vi "ErrorHandling.addLastErrorToFile.vi"(0 "ErrorHandling in":refnum<class "ErrorHandling.lvclass">, 5 "error in (no error)":errorcluster) -> (14 "ErrorHandling out":refnum<class "ErrorHandling.lvclass">, 19 "error out":errorcluster)   [LabVIEW 2016, in "ErrorHandling.lvclass"]
doc: "Schreibt das letzte Error-Ereignis in das entsprechende \"ErrorFile\" gem. System Pfadeintrag\n\n15.04.14 / sige"
uses:
  ErrorHandling.lvclass
  ErrorHandling.lvclass/ErrorHandling.ctl
  <vilib>/dlg_ctls.llb/Space Constant.vi
  <vilib>/Utility/error.llb/Trim Whitespace.vi
  <vilib>/Utility/error.llb/Search and Replace Pattern.vi
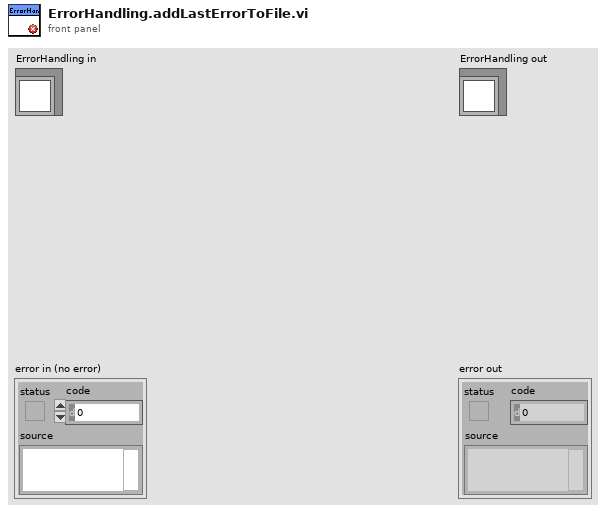
[diagram p1: front panel]
types:
  T1 = enum16{"open", "replace", "create", "open or create", "replace or create", "replace or create with confirmation"}
  T2 = typedef "ErrorHandling.lvclass/ErrorHandling.OccurredErrorDataStruct.ctl" = cluster{"Error":errorcluster, "Caller":string, "Comment":string, "Timestamp":timestamp, "Stopped":bool, "ErrorCusterString":string, "ErrorIndex":u64}
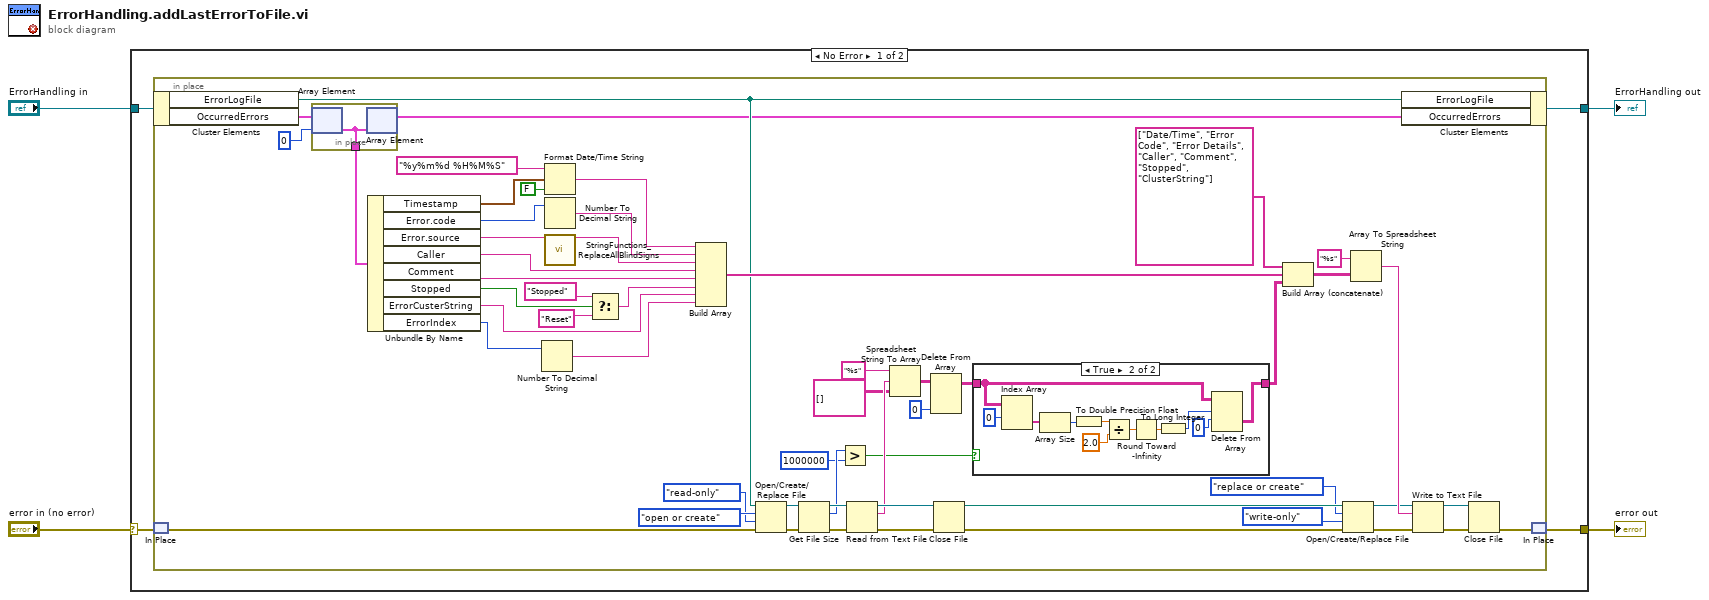
[diagram p0: block diagram]
diagram:
  n1 = case shown="No Error" "error in (no error)" {
    selector: "error in (no error)" -> [w7 w78]
    tunnel: [w6 w78] -> w3
    tunnel: [w5 w77] -> w1
    tunnel: "ErrorHandling in" -> [w8 w77]
    frame No Error {
      n2 = in-place {
        n3 = in-place-cluster #1(w8) -> ("ErrorLogFile"=w13:path, "OccurredErrors"=w12:T2[])
        n4 = in-place-match #2(w7) -> (w15:errorcluster)
        n5 = in-place {
          in-place-border: [w64] -> w11
          n6 = in-place-array #3(w12, 0) -> (w64:T2)
          n7 = in-place-array #3(w64) -> (w10:T2[])  [unwired: 1 out]
        }
        n8 = Unbundle By Name(w11) -> ("Timestamp"=w60:timestamp, "Error.code"=w63:i32, "Error.source"=w21:string, "Caller"=w19:string, "Comment"=w54:string, "Stopped"=w59:bool, "ErrorCusterString"=w18:string, "ErrorIndex"=w17:u64)
        n9 = Number To Decimal String(number=w17) -> (decimal integer string=w16:string)  [unwired: 1 in]
        n10 = Format Date/Time String(time format string (%c)="%y%m%d %H%M%S", seconds (now)=w60, UTC format=FALSE) -> (date/time string=w56:string)
        n11 = Number To Decimal String(number=w63) -> (decimal integer string=w55:string)  [unwired: 1 in]
        n12 = call "StringFunctions_ReplaceAllBlindSigns.vi"("String"=w21) -> ("ModifiedString"=w20:string)  [unwired: 17 in, 1 out]
        n13 = Select(t="Stopped", s=w59, f="Reset") -> (s? t:f=w53:string)
        n14 = Build Array(w56, w55, w20, w19, w54, w53, w18, w16) -> (w36:string[])
        n15 = Open/Create/Replace File(file path (use dialog)=w13, error in=w15, operation (0:open)=T1."open or create", access (0:read/write)=enum16{"read/write", "read-only", "write-only"}."read-only") -> (refnum out=w52:refnum<file>, error out=w46:errorcluster)  [unwired: 2 in, 1 out]
        n16 = Get File Size(file=w52, error in=w46) -> (refnum out=w51:refnum<file>, size (in bytes)=w35:i64, 0:w47:errorcluster)
        n17 = Greater?(x=w35, y=i64 1000000) -> (0:w31:bool)
        n18 = Read from Text File(file (use dialog)=w51, error in=w47) -> (refnum out=w50:refnum<file>, text=w45:string, error out=w28:errorcluster)  [unwired: 2 in, 1 out]
        n19 = Spreadsheet String To Array(format string="%s", spreadsheet string=w45, array type (2D Dbl)=string[][] []) -> (array=w42:string[][])  [unwired: 1 in]
        n20 = Delete From Array(array=w42, index (row)=0) -> (array with subset deleted=w33:string[][])  [unwired: 2 in, 1 out]
        n21 = Close File(refnum=w50, error in=w28) -> (path=w29:path, error out=w26:errorcluster)
        n22 = case shown="True" w31 {
          tunnel: w33 -> [w65 w69]
          tunnel: [w65 w66] -> w32
          frame False {
          }
          frame True {
            n23 = Index Array(array=w69, index (row)=0) -> (element=w75:string[])  [unwired: 1 in]
            n24 = Array Size(array=w75) -> (size(s)=w74:i32)
            n25 = To Double Precision Float(number=w74) -> (double precision float=w72:dbl)
            n26 = Divide(x=w72, y=2.0) -> (x/y=w71:dbl)
            n27 = Round Toward -Infinity(1:w71) -> (0:w70:dbl)
            n28 = To Long Integer(number=w70) -> (32bit integer=w67:i32)
            n29 = Delete From Array(array=w69, length=w67, index (row)=0) -> (deleted portion=w66:string[][])  [unwired: 1 in, 1 out]
          }
        }
        n30 = Build Array (concatenate)(string[] ["Date/Time", "Error Code", "Error Details", "Caller", "Comment", "Stopped", "ClusterString"], w36, w32) -> (w39:string[][])
        n31 = Open/Create/Replace File(file path (use dialog)=w29, error in=w26, operation (0:open)=T1."replace or create", access (0:read/write)=enum16{"read/write", "read-only", "write-only"}."write-only") -> (refnum out=w27:refnum<file>, error out=w25:errorcluster)  [unwired: 2 in, 1 out]
        n32 = Array To Spreadsheet String(array=w39, 3:"%s" ("format string")) -> (spreadsheet string=w37:string)  [unwired: 1 in]
        n33 = in-place-cluster #1("ErrorLogFile"=w13, "OccurredErrors"=w10) -> (w5:refnum<class "ErrorHandling.lvclass">)
        n34 = Write to Text File(file (use dialog)=w27, text=w37, error in=w25) -> (refnum out=w49:refnum<file>, error out=w48:errorcluster)  [unwired: 1 in, 1 out]
        n35 = Close File(refnum=w49, error in=w48) -> (error out=w14:errorcluster)  [unwired: 1 out]
        n36 = in-place-match #2(w14) -> (w6:errorcluster)
      }
    }
    frame Error {
    }
  }
  "error out" <- w3
  "ErrorHandling out" <- w1
